vi "NI9263_driver.vi"(6 "NI9263_method":T1, 8 "error in (no error)":errorcluster, 10 "Variant Values":variant, 11 "Channels NI9263":tag="Dev1/ao0") -> (0 "error out":errorcluster)   [LabVIEW 2020]
uses:
  TYPEDEF/NI9263_TD_Method.ctl
  <vilib>/DAQmx/write.llb/DAQmx Write (Analog 2D DBL NChan NSamp).vi
  <vilib>/DAQmx/write.llb/DAQmx Write (Analog Wfm 1Chan NSamp).vi
  <vilib>/DAQmx/write.llb/DAQmx Write (Analog 1D DBL 1Chan NSamp).vi
  <vilib>/DAQmx/create/channels.llb/DAQmx Create Channel (AO-Voltage-Basic).vi
  <vilib>/DAQmx/configure/timing.llb/DAQmx Timing (Sample Clock).vi
  <vilib>/DAQmx/miscellaneous.llb/DAQmx Fill In Error Info.vi
  <vilib>/DAQmx/configure/timing.llb/DAQmx Timing (Use Waveform).vi
  <vilib>/Utility/Data Type/NI_Data Type.lvlib
  <resource>/objmgr/daqmx.rc
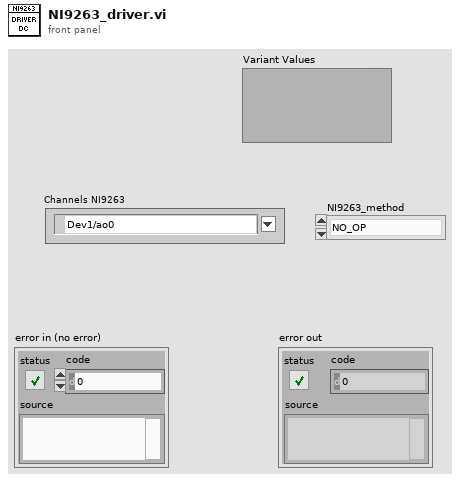
[diagram p1: front panel]
types:
  T1 = typedef "NI9263_TD_Method.ctl" = enum16{"NO_OP", "INIT", "SET", "GET", "CLOSE"}
  T2 = typedef "NI_Data Type.lvlib/Data Type.ctl" = enum8{"Invalid Type", "Void", "I8", "I16", "I32", "I64", "U8", "U16", "U32", "U64", "Single Float", "Double Float", "Extended Float", "Single Complex", "Double Complex", "Extended Complex", "Enum U8", "Enum U16", "Enum U32", "Enum U64", "Single Float With Unit", "Double Float With Unit", "Extended Float With Unit", "Single Complex with Unit", "Double Complex with Unit", "Extended Complex with Unit", "Boolean", "String", "Path", "Picture", "Tag", "Array", "Cluster", "Variant", "LV Variant", "Waveform", "Timestamp", "Digital Waveform", "Digital Data", "ExpressData", "Refnum", "External Data", "VI", "Poly VI", "LabVIEW Class Instance", "Fixed Point", "Set Collection", "Map Collection"}
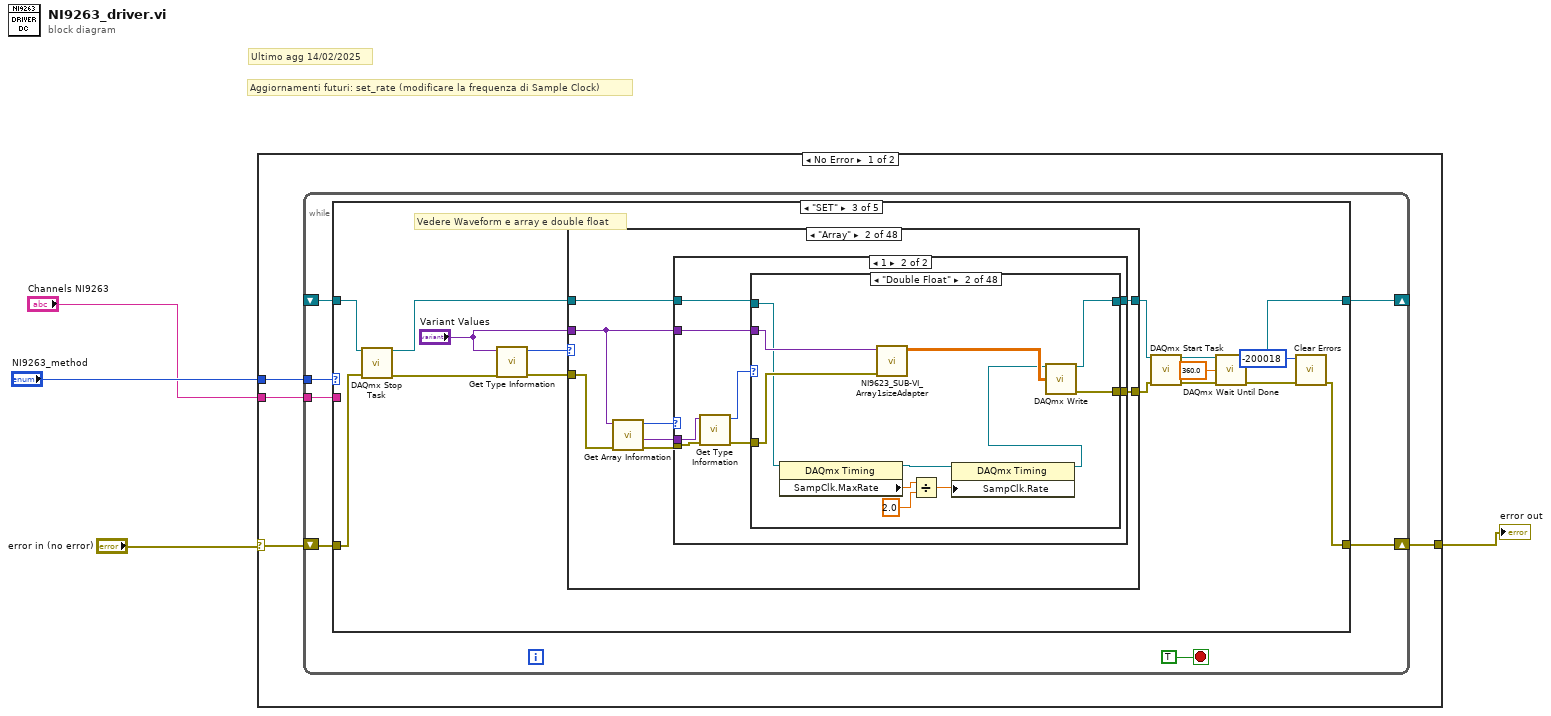
[diagram p0: block diagram]
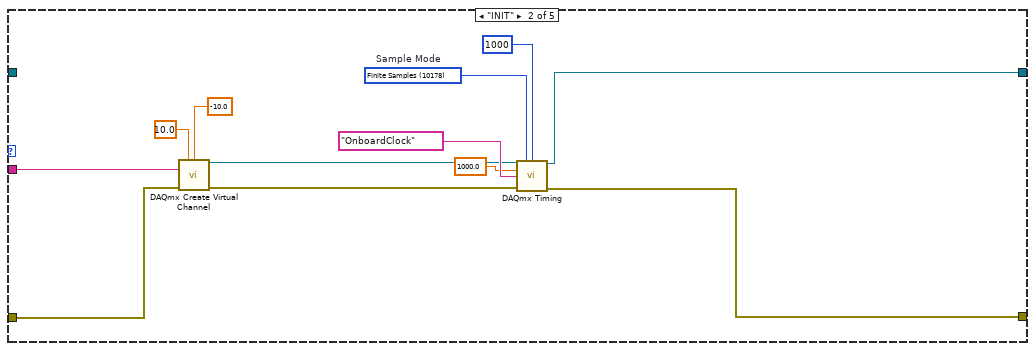
[diagram p3: hidden frame]
diagram:
  # "Aggiornamenti futuri: set_rate (modificare la frequenza di Sample Clock)"
  # "Ultimo agg 14/02/2025"
  n1 = case shown="No Error" "error in (no error)" {
    selector: "error in (no error)" -> [w8 w292]
    tunnel: "NI9263_method" -> [w7 _]
    tunnel: "Channels NI9263" -> [w6 _]
    tunnel: [w5 w292] -> w2
    frame No Error {
      n2 = while {
        tunnel: w7 -> [w14]
        tunnel: w6 -> [w12]
        shift-right: [w11] -> _
        shift-left: _ -> [w10]
        shift-right: [w9] -> w5
        shift-left: w8 -> [w13]
        stop <- TRUE stop-if-true
        n3 = case shown="\"SET\"" w14 {
          tunnel: w13 -> [w16 w27 w36 w284 w286]
          tunnel: w12 -> [_ w26 _ _ _]
          tunnel: [w17 w20 w38 w285 refnum<k21> refnum ("task out")] -> w11
          tunnel: w10 -> [w17 _ w34 w285 w287]
          tunnel: [w16 w21 w31 w284 w289] -> w9
          frame "NO_OP", Default {
          }
          frame "INIT" {
            w25 = 10178 items=["Finite Samples"=10178, "Continuous Samples"=10123, "Hardware Timed Single Point"=12522]  # Sample Mode
            n4 = call-poly <vilib>:"DAQmx Create Virtual Channel.vi"("maximum value"=10.0 ("Max Voltage"), "minimum value"=-10.0 ("Min Voltage"), "physical channels"=w26, "error in"=w27) -> ("task out"=w23:refnum<k21>, "error out"=w22:errorcluster)  [unwired: 10 in]
            n5 = call-poly <vilib>:"DAQmx Timing.vi"("task/channels in"=w23, "sample mode"=w25, "samples per channel"=1000, "rate"=1000.0, "source"=tag "OnboardClock" ("Sample Clock Source"), "error in"=w22) -> ("task out"=w20:refnum<k21>, "error out"=w21:errorcluster)  [unwired: 8 in]
          }
          frame "SET" {
            # "Vedere Waveform e array e double float"
            n6 = call <vilib>:"DAQmx Stop Task.vi"("task/channels in"=w34, "error in"=w36) -> ("task out"=w33:refnum<k21>, "error out"=w35:errorcluster)  [unwired: 12 in]
            n7 = call <vilib>:"Get Type Information.vi"("error in (no error)"=w35, "variant"="Variant Values") -> ("error out"=w44:errorcluster, "type"=w45:T2)  [unwired: 5 in, 3 out]
            n8 = case shown="\"Array\"" w45 {
              tunnel: w44 -> [w46 w52 w171 w173 w175 w185 w188 w190 w192 w194 w196 w198 w200 w202 w204 w206 w208 w210 w212 w214 w216 w218 w220 w222 w224 w226 w228 w230 w235 w246 w248 w250 w252 w254 w256 w258 w260 w262 w264 w266 w268 w270 w272 w274 w276 w278 w280 w282]
              tunnel: [w46 w55 w171 w173 w175 w184 w188 w190 w192 w194 w196 w198 w200 w202 w204 w206 w208 w210 w212 w214 w216 w218 w220 w222 w224 w226 w228 w230 w242 w246 w248 w250 w252 w254 w256 w258 w260 w262 w264 w266 w268 w270 w272 w274 w276 w278 w280 w282] -> w41
              tunnel: [w47 w54 w172 w174 w176 w183 w189 w191 w193 w195 w197 w199 w201 w203 w205 w207 w209 w211 w213 w215 w217 w219 w221 w223 w225 w227 w229 w231 w243 w247 w249 w251 w253 w255 w257 w259 w261 w263 w265 w267 w269 w271 w273 w275 w277 w279 w281 w283] -> w39
              tunnel: w33 -> [w47 w53 w172 w174 w176 w179 w189 w191 w193 w195 w197 w199 w201 w203 w205 w207 w209 w211 w213 w215 w217 w219 w221 w223 w225 w227 w229 w231 w239 w247 w249 w251 w253 w255 w257 w259 w261 w263 w265 w267 w269 w271 w273 w275 w277 w279 w281 w283]
              tunnel: "Variant Values" -> [_ w49 _ _ _ w187 _ _ _ _ _ _ _ _ _ _ _ _ _ _ _ _ _ _ _ _ _ _ w245 _ _ _ _ _ _ _ _ _ _ _ _ _ _ _ _ _ _ _]
              frame "Invalid Type", Default {
              }
              frame "Array" {
                n9 = call <vilib>:"Get Array Information.vi"("error in (no error)"=w52, "variant"=w49) -> ("error out"=w50:errorcluster, "array element data type"=w48:variant, "number of dimensions"=w51:i32)  [unwired: 6 in, 1 out]
                n10 = case shown="1" w51 {
                  tunnel: [w57 w65] -> w55
                  tunnel: [w56 w64] -> w54
                  tunnel: w53 -> [w56 w63]
                  tunnel: w50 -> [w57 w59]
                  tunnel: w49 -> [_ w62]
                  tunnel: w48 -> [_ w61]
                  frame 0, Default {
                  }
                  frame 1 {
                    n11 = call <vilib>:"Get Type Information.vi"("error in (no error)"=w59, "variant"=w61) -> ("error out"=w58:errorcluster, "type"=w60:T2)  [unwired: 5 in, 3 out]
                    n12 = case shown="\"Double Float\"" w60 {
                      tunnel: [w66 w78 w79 w81 w83 w85 w87 w89 w91 w93 w95 w97 w99 w101 w103 w105 w107 w109 w111 w113 w115 w117 w119 w121 w123 w125 w127 w129 w131 w133 w135 w137 w139 w141 w143 w145 w147 w149 w151 w153 w155 w157 w159 w161 w163 w165 w167 w169] -> w65
                      tunnel: [w67 w77 w80 w82 w84 w86 w88 w90 w92 w94 w96 w98 w100 w102 w104 w106 w108 w110 w112 w114 w116 w118 w120 w122 w124 w126 w128 w130 w132 w134 w136 w138 w140 w142 w144 w146 w148 w150 w152 w154 w156 w158 w160 w162 w164 w166 w168 w170] -> w64
                      tunnel: w63 -> [w67 w69 w80 w82 w84 w86 w88 w90 w92 w94 w96 w98 w100 w102 w104 w106 w108 w110 w112 w114 w116 w118 w120 w122 w124 w126 w128 w130 w132 w134 w136 w138 w140 w142 w144 w146 w148 w150 w152 w154 w156 w158 w160 w162 w164 w166 w168 w170]
                      tunnel: w62 -> [_ w76 _ _ _ _ _ _ _ _ _ _ _ _ _ _ _ _ _ _ _ _ _ _ _ _ _ _ _ _ _ _ _ _ _ _ _ _ _ _ _ _ _ _ _ _ _ _]
                      tunnel: w58 -> [w66 w75 w79 w81 w83 w85 w87 w89 w91 w93 w95 w97 w99 w101 w103 w105 w107 w109 w111 w113 w115 w117 w119 w121 w123 w125 w127 w129 w131 w133 w135 w137 w139 w141 w143 w145 w147 w149 w151 w153 w155 w157 w159 w161 w163 w165 w167 w169]
                      frame "Invalid Type", Default {
                      }
                      frame "Double Float" {
                        n13 = property class="DAQmx Timing"(reference=w69) -> (reference out=w73:refnum<k21>, "SampClk.MaxRate"=w71:dbl)  [unwired: 1 in, 1 out]
                        n14 = call "NI9623_SUB-VI_Array1sizeAdapter.vi"("error in (no error)"=w75, "Channel Values"=w76) -> ("Real 2D Array"=w74:dbl[][])  [unwired: 9 in]
                        n15 = Divide(x=w71, y=2.0) -> (x/y=w72:dbl)
                        n16 = property class="DAQmx Timing"(reference=w73, "SampClk.Rate"=w72) -> (reference out=w68:refnum<k21>)  [unwired: 1 in, 1 out]
                        n17 = call-poly <vilib>:"DAQmx Write.vi"("task/channels in"=w68, "data"=w74) -> ("task out"=w77:refnum<k21>, "error out"=w78:errorcluster)  [unwired: 11 in, 1 out]
                      }
                      frame "Extended Float" {
                      }
                      frame "Single Complex" {
                      }
                      frame "Double Complex" {
                      }
                      frame "Extended Complex" {
                      }
                      frame "Enum U8" {
                      }
                      frame "Enum U16" {
                      }
                      frame "Enum U32" {
                      }
                      frame "Enum U64" {
                      }
                      frame "Single Float With Unit" {
                      }
                      frame "Double Float With Unit" {
                      }
                      frame "Extended Float With Unit" {
                      }
                      frame "Single Complex with Unit" {
                      }
                      frame "Double Complex with Unit" {
                      }
                      frame "Extended Complex with Unit" {
                      }
                      frame "Boolean" {
                      }
                      frame "String" {
                      }
                      frame "Path" {
                      }
                      frame "Picture" {
                      }
                      frame "Tag" {
                      }
                      frame "Array" {
                      }
                      frame "Cluster" {
                      }
                      frame "Variant" {
                      }
                      frame "LV Variant" {
                      }
                      frame "Waveform" {
                      }
                      frame "Timestamp" {
                      }
                      frame "Digital Waveform" {
                      }
                      frame "Digital Data" {
                      }
                      frame "ExpressData" {
                      }
                      frame "Refnum" {
                      }
                      frame "External Data" {
                      }
                      frame "VI" {
                      }
                      frame "Poly VI" {
                      }
                      frame "LabVIEW Class Instance" {
                      }
                      frame "Fixed Point" {
                      }
                      frame "Set Collection" {
                      }
                      frame "Map Collection" {
                      }
                      frame "Void" {
                      }
                      frame "I8" {
                      }
                      frame "I16" {
                      }
                      frame "I32" {
                      }
                      frame "I64" {
                      }
                      frame "U8" {
                      }
                      frame "U16" {
                      }
                      frame "U32" {
                      }
                      frame "U64" {
                      }
                      frame "Single Float" {
                      }
                    }
                  }
                }
              }
              frame "Cluster" {
              }
              frame "Variant" {
              }
              frame "LV Variant" {
              }
              frame "Waveform" {
                w182 = 10178 items=["Finite Samples"=10178, "Continuous Samples"=10123, "Hardware Timed Single Point"=12522]  # Sample Mode
                n18 = Variant To Data(error in=w185, type=waveform(dbl) {"t0"=timestamp(0 s since 1904-01-01), "dt"=1.0, "Y"=[]} ("signal out"), Variant=w187) -> (data=w178:waveform(dbl), error out=w177:errorcluster)
                n19 = call-poly <vilib>:"DAQmx Timing.vi"("task/channels in"=w179, "sample mode"=w182, "waveform"=w178, "error in"=w177) -> ("task out"=w180:refnum<k21>, "error out"=w181:errorcluster)  [unwired: 10 in]
                n20 = call-poly <vilib>:"DAQmx Write.vi"("task/channels in"=w180, "data"=w178, "error in"=w181) -> ("task out"=w183:refnum<k21>, "error out"=w184:errorcluster)  [unwired: 10 in, 1 out]
              }
              frame "Timestamp" {
              }
              frame "Digital Waveform" {
              }
              frame "Digital Data" {
              }
              frame "ExpressData" {
              }
              frame "Refnum" {
              }
              frame "External Data" {
              }
              frame "VI" {
              }
              frame "Poly VI" {
              }
              frame "LabVIEW Class Instance" {
              }
              frame "Fixed Point" {
              }
              frame "Set Collection" {
              }
              frame "Map Collection" {
              }
              frame "Void" {
              }
              frame "I8" {
              }
              frame "I16" {
              }
              frame "I32" {
              }
              frame "I64" {
              }
              frame "U8" {
              }
              frame "U16" {
              }
              frame "U32" {
              }
              frame "U64" {
              }
              frame "Single Float" {
              }
              frame "Double Float" {
                n21 = property class="DAQmx Timing"(reference=w239) -> (reference out=w237:refnum<k21>, "SampClk.MaxRate"=w233:dbl)  [unwired: 1 in, 1 out]
                n22 = Variant To Data(error in=w235, type=0.0, Variant=w245) -> (data=w241:dbl)  [unwired: 1 out]
                n23 = Divide(x=w233, y=2.0) -> (x/y=w234:dbl)
                n24 = property class="DAQmx Timing"(reference=w237, "SampClk.Rate"=w234) -> (reference out=w236:refnum<k21>)  [unwired: 1 in, 1 out]
                n25 = Initialize Array(w241, 2 ("dimension size")) -> (w240:dbl[])
                n26 = call-poly <vilib>:"DAQmx Write.vi"("task/channels in"=w236, "data"=w240) -> ("task out"=w243:refnum<k21>, "error out"=w242:errorcluster)  [unwired: 11 in, 1 out]
              }
              frame "Extended Float" {
              }
              frame "Single Complex" {
              }
              frame "Double Complex" {
              }
              frame "Extended Complex" {
              }
              frame "Enum U8" {
              }
              frame "Enum U16" {
              }
              frame "Enum U32" {
              }
              frame "Enum U64" {
              }
              frame "Single Float With Unit" {
              }
              frame "Double Float With Unit" {
              }
              frame "Extended Float With Unit" {
              }
              frame "Single Complex with Unit" {
              }
              frame "Double Complex with Unit" {
              }
              frame "Extended Complex with Unit" {
              }
              frame "Boolean" {
              }
              frame "String" {
              }
              frame "Path" {
              }
              frame "Picture" {
              }
              frame "Tag" {
              }
            }
            n27 = call <vilib>:"DAQmx Start Task.vi"("task/channels in"=w39, "error in"=w41) -> ("task out"=w42:refnum<k21>, "error out"=w40:errorcluster)  [unwired: 12 in]
            n28 = call <vilib>:"DAQmx Wait Until Done.vi"("task/channels in"=w42, "timeout (sec)"=360.0, "error in"=w40) -> ("task out"=w38:refnum<k21>, "error out"=w32:errorcluster)  [unwired: 11 in]
            n29 = call <vilib>:"Clear Errors.vi"("error in (no error)"=w32, "specific error code to clear (0: all)"=-200018) -> ("error out"=w31:errorcluster)  [unwired: 4 in, 1 out]
          }
          frame "GET" {
          }
          frame "CLOSE" {
            n30 = call <vilib>:"DAQmx Stop Task.vi"("task/channels in"=w287, "error in"=w286) -> ("task out"=w290:refnum<k21>, "error out"=w291:errorcluster)  [unwired: 12 in]
            n31 = call <vilib>:"DAQmx Clear Task.vi"("task in"=w290, "error in"=w291) -> ("error out"=w289:errorcluster)  [unwired: 13 in]
          }
        }
      }
    }
    frame Error {
    }
  }
  "error out" <- w2
